vi "Create Room Service Request.vi"(0 "File Data Manager in":refnum<class "File Data Manager.lvclass">, 5 "Rooms No":string, 7 "Room Service":refnum<class "Room Service Base.lvclass">, 11 "error in (no error)":errorcluster) -> (4 "File Data Manager out":refnum<class "File Data Manager.lvclass">, 15 "error out":errorcluster)   [LabVIEW 2023, in "File Data Manager.lvlib" / "File Data Manager.lvclass"]
uses:
  File Data Manager.lvclass
  Room Service Types/Room Service Base/Room Service Base.lvclass
  File Data Manager.lvclass/File Data Manager.ctl
  <vilib>/Utility/miscctls.llb/LVMapReplaceAction.ctl
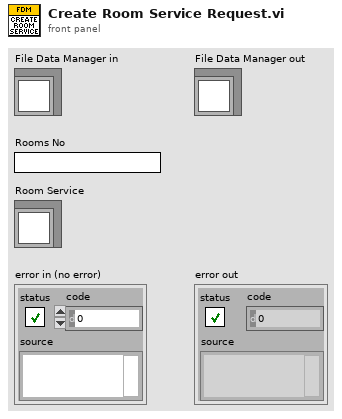
[diagram p1: front panel]
types:
  T1 = typedef "LVMapReplaceAction.ctl" = enum32{"Modify Entry only if found", "Add or Modify Entry", "Delete Entry"}
  T2 = map{string, map{string, refnum<class "Room Service Base.lvclass">}}
  T3 = map{string, refnum<class "Room Service Base.lvclass">}
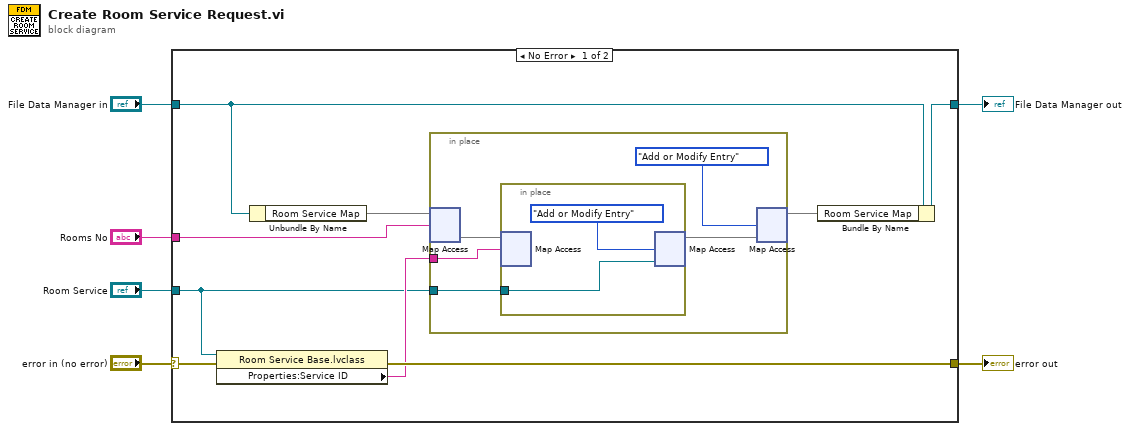
[diagram p0: block diagram]
diagram:
  n1 = case shown="No Error" "error in (no error)" {
    selector: "error in (no error)" -> [w15 w23]
    tunnel: "File Data Manager in" -> [w14 w24]
    tunnel: "Rooms No" -> [w12 _]
    tunnel: [w11 w23] -> w3
    tunnel: "Room Service" -> [w9 _]
    tunnel: [w8 w24] -> w1
    frame No Error {
      n2 = property class="Room Service Base.lvclass"(reference=w9, error in=w15) -> (error out=w11:errorcluster, "Properties:Service ID"=w10:string)  [unwired: 1 out]
      n3 = Unbundle By Name(w14) -> ("Room Service Map"=w13:T2)
      n4 = in-place {
        in-place-border: w10 -> [w19]
        in-place-border: w9 -> [w17]
        n5 = in-place-map #1(w13, w12) -> (w18:T3)  [unwired: 1 in, 1 out]
        n6 = in-place {
          in-place-border: w17 -> [w21]
          n7 = in-place-map #2(w18, w19) -> ()  [unwired: 1 in, 2 out]
          n8 = in-place-map #2(w21, LVMapReplaceAction."Add or Modify Entry" ("action")) -> (w16:T3)  [unwired: 2 out]
        }
        n9 = in-place-map #1(w16, LVMapReplaceAction."Add or Modify Entry" ("action")) -> (w7:T2)  [unwired: 2 out]
      }
      n10 = Bundle By Name(cluster=w14, "Room Service Map"=w7) -> (w8:refnum<class "File Data Manager.lvclass">)
    }
    frame Error {
    }
  }
  "error out" <- w3
  "File Data Manager out" <- w1
